vi "mlink_connect.vi"(8 "error in (no error)":errorcluster, 11 "IP address":string="10.10.1.1") -> (0 "error out":errorcluster, 3 "connection ID":i32)   [LabVIEW 2009, in "MicroDAQ.lvlib" / "mlink.lvlib"]
doc: "This function connects a host PC with MicroDAQ device at given IP address and port. The created connection uses TCP protocol to exchange data between host and MicroDAQ \ndevice. Default port number is 4343. On success, 0 is returned and a valid connection \ndescriptor is stored in the variable pointed by link pointer. Connector descriptor shall be used for all MLink functions as a link_fd argument."
uses:
  <instrlib>/MicroDAQ/Mlink library wraper/mlink.lvlib
  <instrlib>/MicroDAQ/MLink32.dll
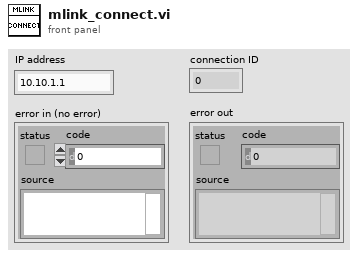
[diagram p1: front panel]
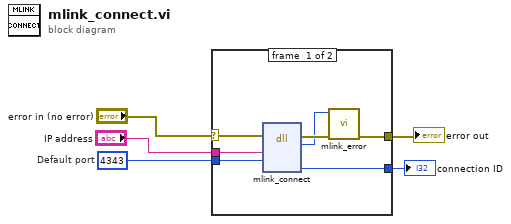
[diagram p0: block diagram]
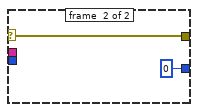
[diagram p2: hidden frame]
diagram:
  w4 = u16 4343  # Default port
  n1 = case shown="No Error" "error in (no error)" {
    selector: "error in (no error)" -> [w7 w14]
    tunnel: [w12 0 ("connection ID")] -> w5
    tunnel: w4 -> [w11 _]
    tunnel: "IP address" -> [w10 _]
    tunnel: [w8 w14] -> w2
    frame #0 {
      n2 = dll-call lib="C:/Program Files (x86)/National Instruments/LabVIEW 2009/instr.lib/MicroDAQ/MLink32.dll" fn="mlink_connect"(error in=w7, "IP address"=w10, "port"=w11) -> (error out=w9:errorcluster, "return type"=w6:i32, "connection ID"=w12:i32)  [unwired: 5 in, 1 out]
      n3 = call <instrlib>:"mlink_error.vi"("error in (no error)"=w9, "error code"=w6) -> ("error out"=w8:errorcluster)  [unwired: 9 in]
    }
    frame #1 {
    }
  }
  "connection ID" <- w5
  "error out" <- w2
